vi "Queque.vi"() -> ()   [LabVIEW 2020]
panel:
  out "Waveform Chart":dbl(graph)
  in  "stop":bool
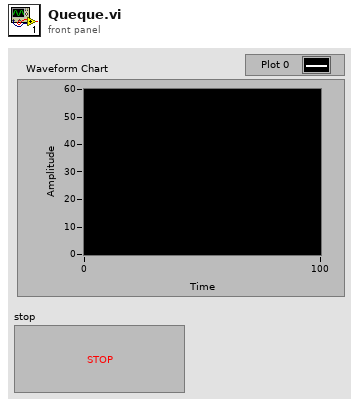
[diagram p1: front panel]
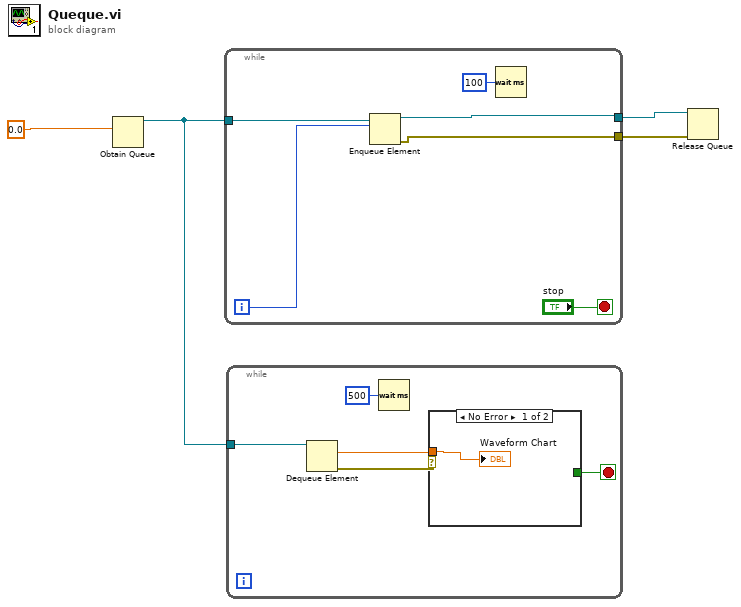
[diagram p0: block diagram]
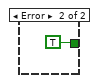
[diagram p2: hidden frame]
diagram:
  n1 = Obtain Queue(element data type=0.0) -> (queue out=w3:refnum<queue>)  [unwired: 4 in, 2 out]
  n2 = while {
    tunnel: w3 -> [w10]
    tunnel: [w7] -> w2
    tunnel: [w6] -> w1
    i -> [w5]
    stop <- "stop" stop-if-true
    n3 = Enqueue Element(queue=w10, element=w5) -> (queue out=w6:refnum<queue>, error out=w7:errorcluster)  [unwired: 2 in, 1 out]
    n4 = Wait (ms)(milliseconds to wait=u32 100) -> ()  [unwired: 1 out]
  }
  n5 = while {
    tunnel: w3 -> [w13]
    stop <- w14 stop-if-true
    n6 = Dequeue Element(queue=w13) -> (element=w11:dbl, error out=w12:errorcluster)  [unwired: 2 in, 2 out]
    n7 = Wait (ms)(milliseconds to wait=u32 500) -> ()  [unwired: 1 out]
    n8 = case shown="No Error" w12 {
      tunnel: [_ TRUE] -> w14
      tunnel: w11 -> [w16 _]
      frame No Error {
        "Waveform Chart" <- w16
      }
      frame Error {
      }
    }
  }
  n9 = Release Queue(queue=w1, error in (no error)=w2) -> ()  [unwired: 1 in, 3 out]
